vi "Read Actors to Nest.vi"(11 "Template in":refnum<class "Template.lvclass">) -> (3 "Actors to Nest":refnum<class "Actor.lvclass">[](array[class]))   [LabVIEW 2020, in "Template.lvlib" / "Template.lvclass"]
doc: "Returns the actors to nest array"
uses:
  Template.lvclass
  <vilib>/ActorFramework/Actor/Actor.lvclass
  Template.lvclass/Template.ctl
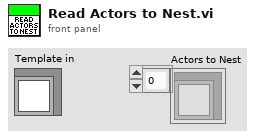
[diagram p1: front panel]
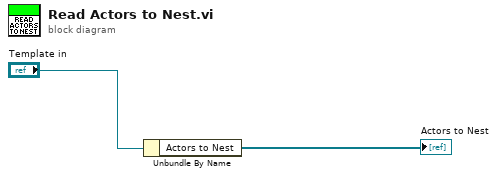
[diagram p0: block diagram]
diagram:
  n1 = Unbundle By Name("Template in") -> ("Actors to Nest"=→"Actors to Nest":refnum<class "Actor.lvclass">[])
